vi "SubVI_LR_Cclock.vi"(9 "Left":dbl(slide) scale=1.0..-1.0, 10 "Forward":dbl(slide) scale=-1.0..1.0) -> (1 "CounterClock":dbl(slide) scale=1.0..-1.0, 2 "Forward":dbl(slide) scale=-1.0..1.0)   [LabVIEW 2017]
panel:
  # "Input (percentage)"
  # "Out (after limiting)"
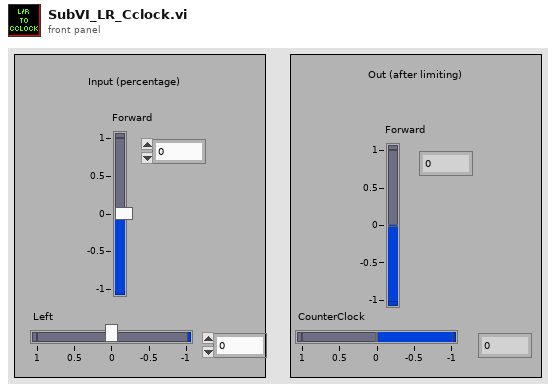
[diagram p1: front panel]
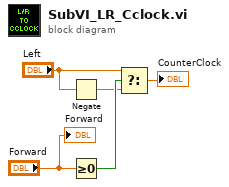
[diagram p0: block diagram]
diagram:
  n1 = Negate(x="Left") -> (-x=w1:dbl)
  n2 = Greater Or Equal To 0?(x="Forward") -> (x >= 0?=w4:bool)
  n3 = Select(t="Left", s=w4, f=w1) -> (s? t:f=→"CounterClock":dbl)
  "Forward" <- "Forward"
